vi "Dashboard Main.vi"() -> ()   [LabVIEW 2015]
uses:
  <vilib>/Utility/miscctls.llb/LVRowAndColumnTypeDef.ctl
  <vilib>/event_ctls.llb/eventvkey.ctl
  <vilib>/Rock Robotics/WPI/Dashboard/WPI_DashboardLogging Global.vi
  <vilib>/Rock Robotics/Network Tables/NT Read Numeric Array.vi
  <vilib>/Utility/config.llb/Write Key (String).vi
  <vilib>/Utility/config.llb/Write Key (I32).vi
  <vilib>/Utility/config.llb/NI_LVConfig.lvlib
panel:
  in  "TCP":refnum<k5>
  in  "Rec Mode":enum32{"Stop", "Record", "Playback"}(radio)
  in  "Vision":u16(ring) items=["Camera Off", "USB Camera SW", "USB Camera HW", "IP Camera"]
  out "Camera IP":string
  out "Image Message":string="Timeout in Camera Communications"
  in  "Dashboard Tab":T1(tab)
  out "String":string
  in  "Select Auto":string(combo)
  out "NT Connection":bool
  in  "Camera Settings":T2={"Frame Rate"=30, "Compression"=30, "Size"=1} {"Frame Rate" scale=1.0..30.0; "Size" items=["640x480", "320x240", "160x120"]}
  out "MotorChart R":cluster{"Numeric":dbl, "Numeric":dbl}(graph)
  out "MotorChart L":T3(graph)
  out "MotorSliders R":cluster{"MotorSlide1":dbl, "MotorSlide2":dbl} {"MotorSlide2" scale=-1.0..1.0 scale format="%#_2e"; "MotorSlide1" scale=-1.0..1.0 scale format="%#_2e"}
  out "MotorSliders L":T4 {"MotorSlide4 2" scale=0.0..14.0 scale format="%#_2e"; "MotorSlide2" scale=-1.0..1.0 scale format="%#_2e"; "MotorSlide1" scale=-1.0..1.0 scale format="%#_2e"}
  out "Gyro":dbl(knob) scale=0.0..360.0
  out "JS1 Z":dbl(slide) scale=-1.0..1.0 scale format="%#_2e"
  out "JS1 Graph":cluster{"X":dbl, "Y":dbl}[](graph)
  out "JS1 Buttons":T5
  out "JS2 Z":dbl(slide) scale=-1.0..1.0 scale format="%#_2e"
  out "JS2 Graph":cluster{"X":dbl, "Y":dbl}[](graph)
  out "JS2 Buttons":T5
  out "Mode":T6(ring)=enum."Auto Disabled"
  in  "DB Camera Config":bool
  out "fps":dbl format="%#.1g"
  out "Mbps":dbl format="%#.1g"
  out "Mbps LED":bool
  in  "Numeric":dbl
  in  "DB/String 9":string
  in  "DB/String 8":string
  in  "DB/String 7":string
  in  "DB/String 6":string
  in  "DB/String 5":string
  in  "DB/String 4":string
  in  "DB/String 3":string
  in  "DB/String 2":string
  in  "DB/String 1":string
  in  "DB/String 0":string
  in  "DB/Slider 0":dbl(slide) scale=0.0..5.0
  in  "DB/Slider 1":dbl(slide) scale=0.0..5.0
  in  "DB/Slider 2":dbl(slide) scale=0.0..5.0
  in  "DB/Slider 3":dbl(slide) scale=0.0..5.0
  out "DB/LED 3":bool
  out "DB/LED 2":bool
  out "DB/LED 1":bool
  out "DB/LED 0":bool
  in  "DB/Button 3":bool
  in  "DB/Button 2":bool
  in  "DB/Button 1":bool
  in  "DB/Button 0":bool caption="New Name"
  out "Gyro":dbl
  out "Sonar":dbl
  out "Gyro 2":dbl
  in  "Test Slider":dbl(slide) scale=0.0..100.0 scale format="%#_3g"
  in  "On/Off":bool caption="Solenoid"
  in  "Test Name":u16(ring) items=["Select the test to run..."]
  in  "Test Tree":string(tree)
  in  "Motor":cluster{"Value":dbl, "Enable":bool} {"Value" scale=-1.0..1.0 scale format="%#_3g"}
  out "Progress":T7 {"Test Progress" scale=0.0..100.0}
  in  "Rev/Fwd":cluster{"Forward":bool, "Reverse":bool}
  in  "Test Ring":u16(ring) items=["Monochrome", "Color"]
  out "Cmd Status":string
  in  "Execute Command":bool
  in  "Command Params":string[][](table)
  in  "Command Selection":i32(listbox)
  in  "CheckList":i32(listbox)
  out "Tree":string(tree)
  out "Camera Image":T8(plugin-control)
  out "Background":bool
  # "Left"
  # "Front"
  # "Right"
  # "Battery"
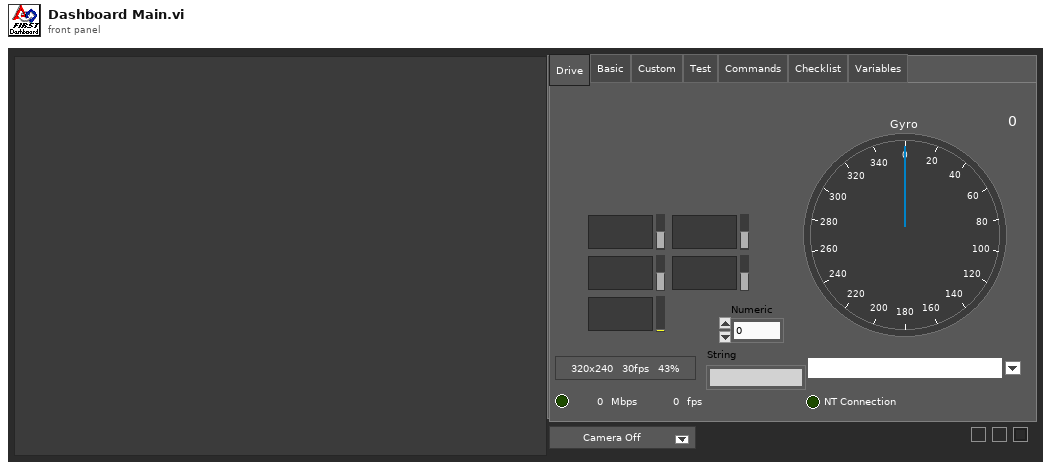
[diagram p1: front panel]
types:
  T1 = enum32{"Drive", "Basic", "Custom", "Test", "Commands", "Checklist", "Variables"}
  T2 = cluster{"Frame Rate":i32, "Compression":i32, "Size":u16}
  T3 = cluster{"Numeric":dbl, "Numeric":dbl, "Battery V":dbl}
  T4 = cluster{"MotorSlide1":dbl, "MotorSlide2":dbl, "MotorSlide4 2":dbl}
  T5 = cluster{bool, bool, bool, bool, bool, bool, bool, bool, bool, bool, bool, bool}
  T6 = enum8{"Tele-Op Disabled", "Tele-Op Enabled", "Auto Disabled", "Auto Enabled", "Test Disabled", "Test Enabled", "Disconnected", "No Code", "E-Stop"}
  T7 = cluster{"Test Progress":u8, "Test Progress Text":string}
  T8 = typedef "IMAQ Image.ctl" = refnum<image>
  T9 = cluster{"IDs":cluster{"RPC field ID":u16, "Unique ID":u16}, "String":string}
  T10 = enum32{"Drive", "Basic", "Custom", "Test", "Checklist", "Variables"}
  T11 = typedef "Image Type" = u32
  T12 = cluster{"Camera Image":refnum<vi>, "Dashboard Tab":refnum<vi>, "Background":refnum<vi>, "Vision":refnum<vi>, "Rec Mode":refnum<vi>, "Test Slider":refnum<vi>, "On/Off ":refnum<vi>, "Test Ring":refnum<vi>, "Rev/Fwd":refnum<vi>, "Test Name":refnum<vi>, "Motor":refnum<vi>, "Progress":refnum<vi>, "CheckList":refnum<vi>, "Tree":refnum<vi>, "Test Tree":refnum<vi>, "Command Params":refnum<vi>, "Command Selection":refnum<vi>, "Execute Command":refnum<vi>, "Cmd Status":refnum<vi>}
  T13 = cluster{"Error Strings":string, "Disable Counts":cluster{u16, u16}, "Rail Faults":cluster{u16, u16, u16}, "Robot IP":string, "DB Mode":u8, "Event Info":cluster{"Name":string, "Type":u8, "Number":u16, "Replay":u8}, "Camera Addr":string}
  T14 = cluster{"Storage":cluster{"Disk Free":u64, "RAM Block":u32, "RAM free":u32}, "CPU Utilization":cluster{"CPU % ISR":sgl, "CPU % Time Crit":sgl, "CPU % Timed Str":sgl, "CPU % High":sgl, "CPU % Above":sgl, "CPU % Normal":sgl, "CPU % Low":sgl}, "CAN":cluster{"% Bus Utilization":sgl, "Bus Off Cnt":u32, "TX_FIFO Full Cnt":u32, "Receive Error Cnt":u8, "Transmit Error Cnt":u8}, "HID":cluster{"HID Outputs":u32, "Rumble Low":u16, "Rumble High":u16}[]}
  T15 = cluster{"Status bits":cluster{"Test Mode":bool, "Autonomous":bool, "Enabled":bool, "Code Start":bool, "Brownout":bool, "Reserved 2":bool, "Reserved 3":bool, "E-Stop":bool}, "Code Trace":cluster{"Disabled":bool, "TeleOp":bool, "Auto":bool, "Test":bool}, "Controller Type":enum16{"unknown", "cRIO", "roboRio"}, "Code?":enum16{"unknown", "noCode", "code"}, "Battery V":dbl}
  T16 = cluster{"Control Bits":cluster{"TestMode":bool, "Autonomous":bool, "Enabled":bool, "FMS Present":bool, bool, bool, bool, "E-Stop":bool}, "Team Station ":u8, "Countdown":sgl, "Joystick Values":cluster{"Axes":dbl[], "Buttons":bool[], "POVs":i16[]}[]}
  T17 = cluster{"Axes":dbl[], "Buttons":bool[], "POVs":i16[]}[]
  T18 = cluster{"Axes":dbl[], "Buttons":bool[], "POVs":i16[]}
  T19 = cluster{"Buttons[0]":bool, "Buttons[1]":bool, "Buttons[2]":bool, "Buttons[3]":bool, "Buttons[4]":bool, "Buttons[5]":bool, "Buttons[6]":bool, "Buttons[7]":bool, "Buttons[8]":bool, "Buttons[9]":bool, "Buttons[10]":bool, "Buttons[11]":bool}
  T20 = cluster{"Desired Font (Application)":enum16{"User-specified Font", "Application Font", "System Font", "Dialog Font"}, "[User-specified Font]":cluster{"Font Name":string, "Size":i16, "Strikeout?":bool, "Italic?":bool, "Underline?":bool, "Outline?":bool, "Shadow?":bool, "Bold?":bool, "Rotation Angle":dbl}, "Horizontal Alignment":i16, "Vertical Alignment":i16}
  T21 = typedef "NI_LVConfig.lvlib/Config Data RefNum.ctl" = refnum<k1>
  T22 = cluster{"Operation":enum16{"Update", "Clear"}, "Color Box":u32}[]
  T23 = typedef "eventvkey.ctl" = enum16{"ASCII", "Enter", "Return", "Shift", "Ctrl", "Alt", "Cmd", "Opt", "Caps", "NumLock", "Clear", "Break", "Up", "Down", "Left", "Right", "Insert", "Delete", "Home", "End", "PageUp", "PageDown", "Escape", "Help", "Pause", "ScrollLock", "F1", "F2", "F3", "F4", "F5", "F6", "F7", "F8", "F9", "F10", "F11", "F12", "F13", "F14", "F15", "F16", "F17", "F18", "F19", "F20", "F21", "F22", "F23", "F24", "Play", "VolumeUp", "VolumeDown", "Mute", "Two Byte Char"}
  T24 = cluster{"Image Size":bool, "Image Type":bool, "Pixel Value":bool, "ROI Information":bool, "Zoom Factor":bool}
  T25 = enum8{"Enabled", "Disabled", "Disabled and Grayed Out"}
  T26 = cluster{"Operation":enum16{"Update", "Clear"}, "Color Box":u32}
  T27 = typedef "LVRowAndColumnTypeDef.ctl" = cluster{"Row":i32, "Column":i32}
  T28 = cluster{"Shift":bool, "Ctrl":bool, "Alt":bool, "Cmd":bool, "Opt":bool}
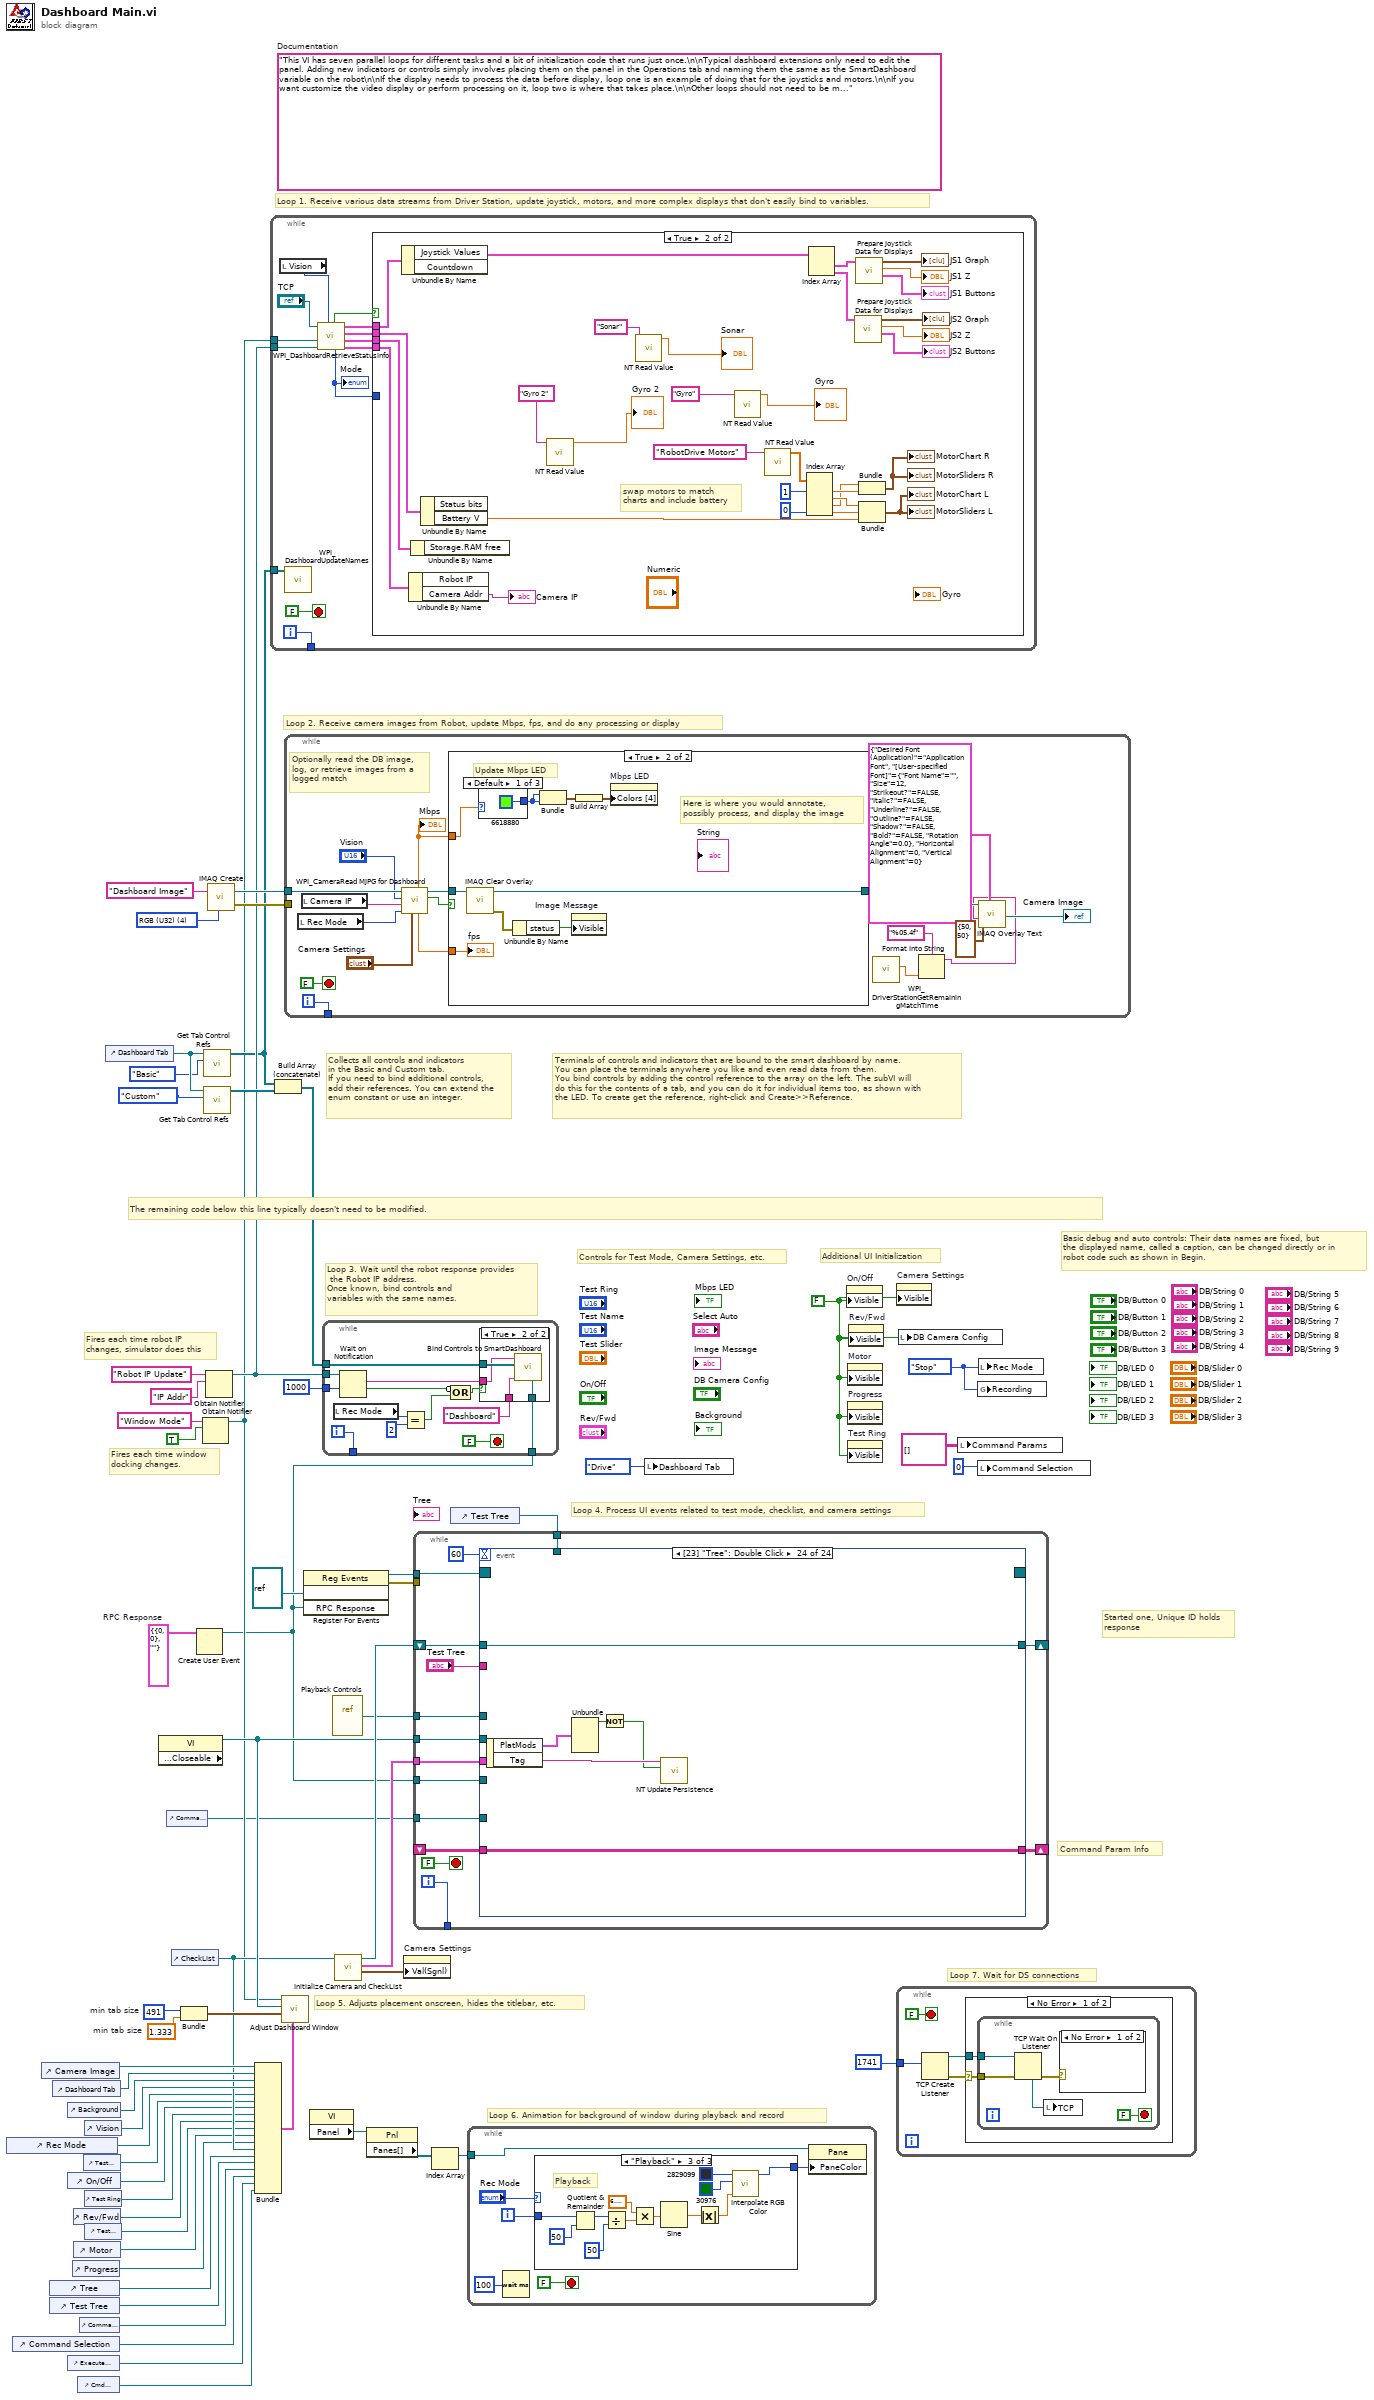
[diagram p0: block diagram]
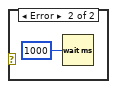
[diagram p2: hidden frame]
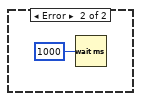
[diagram p3: hidden frame]
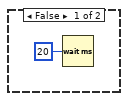
[diagram p4: hidden frame]
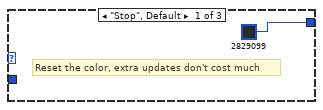
[diagram p5: hidden frame]
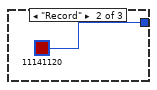
[diagram p6: hidden frame]
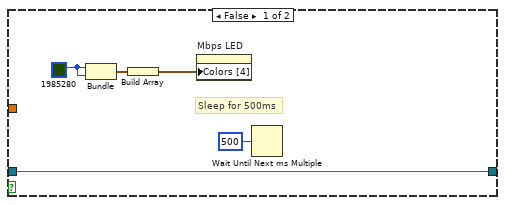
[diagram p8: hidden frame]
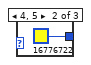
[diagram p9: hidden frame]
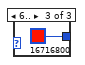
[diagram p10: hidden frame]
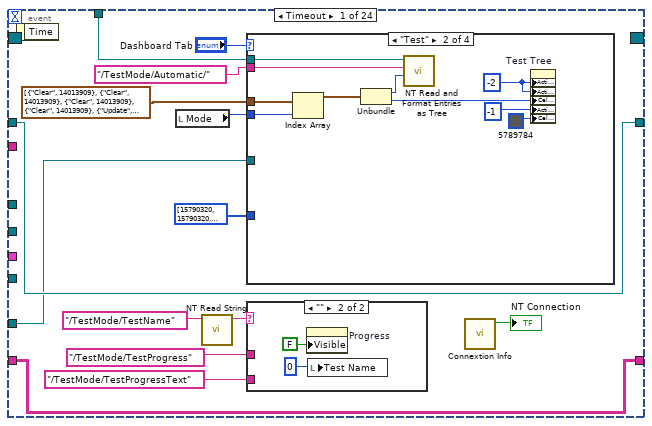
[diagram p11: hidden frame]
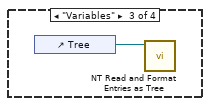
[diagram p13: hidden frame]
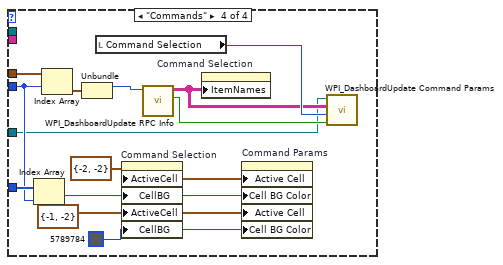
[diagram p14: hidden frame]
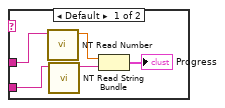
[diagram p15: hidden frame]
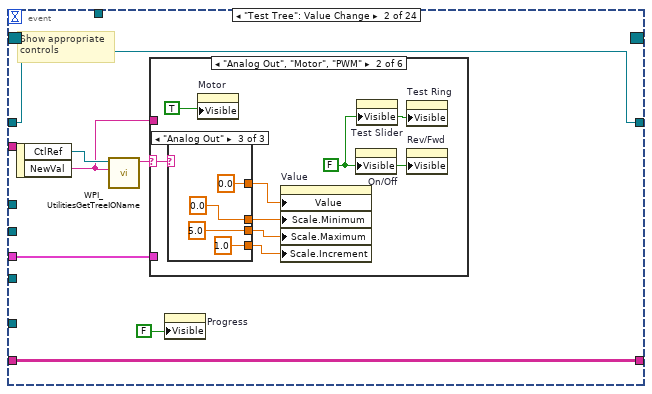
[diagram p16: hidden frame]
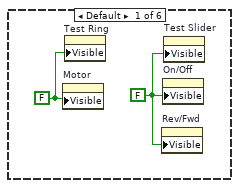
[diagram p17: hidden frame]
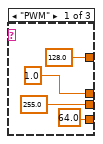
[diagram p18: hidden frame]
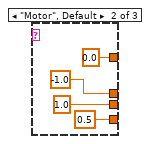
[diagram p19: hidden frame]
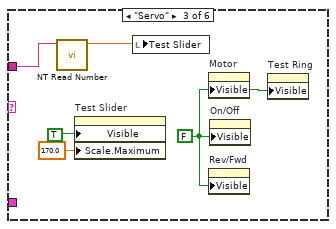
[diagram p20: hidden frame]
diagram:
  w7 = T9 {"IDs"={"RPC field ID"=0, "Unique ID"=0}, "String"=""}  # RPC Response
  w33 = 491  # min tab size
  w32 = 1.333  # min tab size
  w41 = enum32{"Stop", "Record", "Playback"}."Stop" ("Rec Mode")
  w15 = FALSE ("Visible")
  (unwired) "This VI has seven parallel loops for different tasks and a bit of initialization code that runs just once.\n\nTypical dashboard extensions only need to edit the panel. Adding new indicators or controls simply involves placing them on the panel in the Operations tab and naming them the same as the SmartDashboard variable on the robot\n\nIf the display needs to process the data before display, loop one is an example of doing that for the joysticks and motors.\n\nIf you want customize the video display or perform processing on it, loop two is where that takes place.\n\nOther loops should not need to be modified. They are pretty standard, and document the task they perform."  # Documentation
  w61 = T11 4 items=["Grayscale (U8)", "Grayscale (I16)", "Grayscale (SGL)", "Complex (CSG)", "RGB (U32)", "HSL (U32)", "RGB (U64)"] ("Image Type")
  # "Command Param Info"
  # "Started one, Unique ID holds\nresponse"
  # "Loop 7. Wait for DS connections"
  # "Basic debug and auto controls: Their data names are fixed, but\nthe displayed name, called a caption, can be changed directly or in\nrobot code such as shown in Begin."
  # "Controls for Test Mode, Camera Settings, etc."
  # "Additional UI Initialization"
  # "Loop 6. Animation for background of window during playback and record"
  # "Fires each time robot IP\nchanges, simulator does this"
  # "Fires each time window\ndocking changes."
  # "Collects all controls and indicators\nin the Basic and Custom tab.\nIf you need to bind additional controls,\nadd their references. You can extend the\nenum constant or use an integer."
  # "The remaining code below this line typically doesn't need to be modified."
  # "Loop 4. Process UI events related to test mode, checklist, and camera settings"
  # "Terminals of controls and indicators that are bound to the smart dashboard by name.\nYou can place the terminals anywhere you like and even read data from them.\nYou bind controls by adding the control reference to the array on the left. The subVI will\ndo this for the contents of a tab, and you can do it for individual items too, as shown with\nthe LED. To create get the reference, right-click and Create>>Reference."
  # "Loop 3. Wait until the robot response provides\n the Robot IP address.\nOnce known, bind controls and\nvariables with the same names."
  # "Loop 5. Adjusts placement onscreen, hides the titlebar, etc."
  # "Loop 1. Receive various data streams from Driver Station, update joystick, motors, and more complex displays that don't easily bind to variables."
  # "Loop 2. Receive camera images from Robot, update Mbps, fps, and do any processing or display"
  n1 = control-ref of="Rec Mode"() -> (w21:refnum<vi>)
  n2 = control-ref of="Command Selection"() -> (w6:refnum<vi>)
  n3 = control-ref of="Camera Image"() -> (w36:refnum<vi>)
  n4 = control-ref of="Tree"() -> (w25:refnum<vi>)
  n5 = control-ref of="Test Tree"() -> (w24:refnum<vi>)
  n6 = control-ref of="Dashboard Tab"() -> (w35:refnum<vi>)
  n7 = control-ref of="Execute Command"() -> (w8:refnum<vi>)
  n8 = control-ref of="Background"() -> (w30:refnum<vi>)
  n9 = control-ref of="On/Off"() -> (w19:refnum<vi>)
  n10 = control-ref of="Progress"() -> (w16:refnum<vi>)
  n11 = control-ref of="Rev/Fwd"() -> (w17:refnum<vi>)
  n12 = control-ref of="Motor"() -> (w22:refnum<vi>)
  n13 = control-ref of="Cmd Status"() -> (w2:refnum<vi>)
  n14 = control-ref of="Command Params"() -> (w9:refnum<vi>)
  n15 = control-ref of="Test Slider"() -> (w20:refnum<vi>)
  n16 = control-ref of="Vision"() -> (w34:refnum<vi>)
  n17 = control-ref of="Test Ring"() -> (w18:refnum<vi>)
  n18 = control-ref of="Test Name"() -> (w23:refnum<vi>)
  n19 = control-ref of="Dashboard Tab"() -> (w39:refnum<vi>)
  n20 = property class="VI" props=["Front Panel.Closeable"]() -> (reference out=w40:refnum<vi>)  [unwired: 2 in, 2 out]
  n21 = control-ref of="Command Params"() -> (w1:refnum<vi>)
  n22 = control-ref of="CheckList"() -> (w26:refnum<vi>)
  n23 = Bundle("min tab size"=w33, "min tab size"=w32) -> (w31:cluster{"min tab size":i32, "min tab size":dbl})  [unwired: 1 in]
  n24 = Create User Event(user event datatype=w7) -> (user event=w3:refnum<user-event>)  [unwired: 1 in, 1 out]
  n25 = Obtain Notifier(name (unnamed)="Window Mode", notification data type=TRUE) -> (notifier out=w12:refnum<notifier>)  [unwired: 2 in, 2 out]
  n26 = call <vilib>:"Get Tab Control Refs.vi"("Page Index"=T10."Basic" ("Dashboard Tab"), "TabControl in"=w39) -> ("ControlsOnPage"=w13:refnum<vi>[])  [unwired: 9 in]
  n27 = call <vilib>:"Get Tab Control Refs.vi"("Page Index"=T10."Custom" ("Dashboard Tab"), "TabControl in"=w39) -> ("ControlsOnPage"=w38:refnum<vi>[])  [unwired: 9 in]
  n28 = Obtain Notifier(name (unnamed)="Robot IP Update", notification data type="IP Addr" ("name (unnamed)")) -> (notifier out=w14:refnum<notifier>)  [unwired: 2 in, 2 out]
  n29 = call "IMAQ Create"("Image Name"="Dashboard Image", "Image Type"=w61) -> ("New Image"=w59:T8, "error out"=w58:errorcluster)  [unwired: 2 in, 1 out]
  n30 = Bundle("Camera Image"=w36, "Dashboard Tab"=w35, "Background"=w30, "Vision"=w34, "Rec Mode"=w21, "Test Slider"=w20, "On/Off"=w19, "Test Ring"=w18, "Rev/Fwd"=w17, "Test Name"=w23, "Motor"=w22, "Progress"=w16, "CheckList"=w26, "Tree"=w25, "Test Tree"=w24, "Command Params"=w9, "Command Selection"=w6, "Execute Command"=w8, "Cmd Status"=w2) -> (w27:T12)  [unwired: 1 in]
  n31 = while {
    tunnel: [w73] -> _
    tunnel: w14 -> [w67]
    tunnel: w13 -> [w66]
    tunnel: w12 -> [w62]
    i -> [w73]
    stop <- FALSE stop-if-true
    n32 = local read "Vision"() -> (w64:u16)
    n33 = call <vilib>:"WPI_DashboardUpdateNames.vi"("Controls on Tab"=w66) -> ()  [unwired: 11 in]
    n34 = call <vilib>:"WPI_DashboardRetrieveStatusInfo.vi"("Vision"=w64, "Binding Refnum"=w67, "Window Mode Notifier"=w62, "TCP Cnx"="TCP") -> ("Power and Errors"=w68:T13, "Robot Metrics"=w71:T14, "Status Info"=w72:T15, "Control Info"=w69:T16, "Robot Mode"=w65:T6, "Process?"=w70:bool)  [unwired: 2 in]
    "Mode" <- w65
    n35 = case shown="True" w70 {
      tunnel: w72 -> [_ w106]
      tunnel: w71 -> [_ w105]
      tunnel: w69 -> [_ w104]
      tunnel: w68 -> [_ w103]
      tunnel: w65 -> [_ _]
      frame False {
        n36 = Wait (ms)(milliseconds to wait=u32 20) -> ()  [unwired: 1 out]
      }
      frame True {
        # "swap motors to match\ncharts and include battery"
        n37 = Unbundle By Name(w104) -> ("Joystick Values"=w93:T17)  [unwired: 1 out]
        n38 = Unbundle By Name(w103) -> ("Camera Addr"=→"Camera IP":string)  [unwired: 1 out]
        n39 = Unbundle By Name(w105) -> ()  [unwired: 1 out]
        n40 = Unbundle By Name(w106) -> ("Battery V"=w94:dbl)  [unwired: 1 out]
        n41 = call-poly <vilib>:"NT Read Value.vi"("Name"="Gyro 2") -> ("Numeric"=→"Gyro 2":dbl)  [unwired: 9 in, 1 out]
        n42 = call-poly <vilib>:"NT Read Value.vi"("Name"="Sonar") -> ("Numeric"=→"Sonar":dbl)  [unwired: 9 in, 1 out]
        n43 = call-poly <vilib>:"NT Read Value.vi"("Name"="Gyro") -> ("Numeric"=→"Gyro":dbl)  [unwired: 9 in, 1 out]
        n44 = call-poly <vilib>:"NT Read Value.vi"("Name"="RobotDrive Motors") -> ("Numeric Array"=w82:dbl[])  [unwired: 9 in, 1 out]
        n45 = Index Array(array=w82, index #1=1, index #4=0) -> (element #1=w98:dbl, element #2=w99:dbl, element #3=w97:dbl, element #4=w102:dbl)  [unwired: 2 in]
        n46 = Index Array(array=w93) -> (element #1=w92:T18, element #2=w87:T18)  [unwired: 2 in]
        n47 = call "Prepare Joystick Data for Displays.vi"("Joystick Values"=w87) -> ("Buttons"=→"JS2 Buttons":T19, "Z Axis"=→"JS2 Z":dbl, "Cartesian Data"=→"JS2 Graph":cluster{"X axis":dbl, "X axis":dbl}[])  [unwired: 8 in]
        n48 = call "Prepare Joystick Data for Displays.vi"("Joystick Values"=w92) -> ("Buttons"=→"JS1 Buttons":T19, "Z Axis"=→"JS1 Z":dbl, "Cartesian Data"=→"JS1 Graph":cluster{"X axis":dbl, "X axis":dbl}[])  [unwired: 8 in]
        n49 = Bundle("Numeric"=w97, "Numeric"=w98) -> (→"MotorChart R" →"MotorSliders R":cluster{"Numeric":dbl, "Numeric":dbl})  [unwired: 1 in]
        n50 = Bundle("Numeric"=w99, "Numeric"=w102, "Battery V"=w94) -> (→"MotorChart L" →"MotorSliders L":T3)  [unwired: 1 in]
      }
    }
  }
  n51 = Build Array (concatenate)(w13, w38) -> (w37:refnum<vi>[])
  n52 = call "Adjust Dashboard Window.vi"("Sizing Refnums"=w27, "Size Constraints"=w31, "VI"=w40, "WIn Mode"=w12) -> ()  [unwired: 8 in]
  n53 = while {
    tunnel: w59 -> [w122]
    tunnel: w58 -> [_]
    tunnel: [w123] -> _
    i -> [w123]
    stop <- FALSE stop-if-true
    # "Optionally read the DB image,\nlog, or retrieve images from a\nlogged match"
    n54 = local read "Rec Mode"() -> (w117:enum32{"Stop", "Record", "Playback"})
    n55 = local read "Camera IP"() -> (w115:string)
    n56 = call <vilib>:"WPI_CameraRead MJPG for Dashboard.vi"("Camera Settings"="Camera Settings", "Rec Mode"=w117, "Camera IP"=w115, "Camera Mode"="Vision", "Refnum in"=w122) -> ("Active"=w120:bool, "Refnum out"=w121:T8, "FPS"=w119:dbl, "Bandwidth (Mbps)"=w114:dbl)  [unwired: 3 in]
    "Mbps" <- w114
    n57 = case shown="True" w120 {
      tunnel: w121 -> [w125 w133]
      tunnel: w114 -> [_ w132]
      tunnel: w119 -> [_ w131]
      tunnel: [w125 w130] -> w113
      frame False {
        w126 = u32 1985280 ("Color Box")
        # "Sleep for 500ms"
        n58 = Bundle("Color Box"=w126, "Color Box"=w126) -> (w128:cluster{"Color Box":u32, "Color Box":u32})  [unwired: 1 out]
        n59 = Build Array(w128) -> (w127:cluster{"Color Box":u32, "Color Box":u32}[])
        n60 = property on="Mbps LED" class="Bool (strict)"("Colors [4]"=w127) -> ()  [unwired: 2 in, 2 out]
        n61 = Wait Until Next ms Multiple(millisecond multiple=u32 500) -> ()  [unwired: 1 out]
      }
      frame True {
        # "Here is where you would annotate,\npossibly process, and display the image"
        # "Update Mbps LED"
        n62 = call "IMAQ Clear Overlay"("Image"=w133) -> ("error out"=w137:errorcluster, "Image Out"=w130:T8)  [unwired: 2 in, 7 out]
        n63 = case shown="Default" w132 {
          tunnel: [u32 6618880 ("Color Box") u32 16776722 ("Color Box") u32 16716800 ("Color Box")] -> w134
          frame Default {
          }
          frame 4, 5 {
          }
          frame 6.. {
          }
        }
        n64 = Unbundle By Name(w137) -> ("status"=w138:bool)
        n65 = Bundle("Color Box"=w134, "Color Box"=w134) -> (w136:cluster{"Color Box":u32, "Color Box":u32})  [unwired: 1 out]
        n66 = property on="Image Message" class="Str"("Visible"=w138) -> ()  [unwired: 2 in, 2 out]
        n67 = Build Array(w136) -> (w135:cluster{"Color Box":u32, "Color Box":u32}[])
        n68 = property on="Mbps LED" class="Bool (strict)"("Colors [4]"=w135) -> ()  [unwired: 2 in, 2 out]
        "fps" <- w131
      }
    }
    n69 = call <vilib>:"WPI_DriverStationGetRemainingMatchTime.vi"() -> ("Match Time(s)"=w109:sgl)  [unwired: 10 in, 1 out]
    n70 = Format Into String(format string="%05.4f", w109) -> (resulting string=w108:string)  [unwired: 2 in, 1 out]
    n71 = call "IMAQ Overlay Text"("Font, Size & Style"=T20 {"Desired Font (Application)"=enum."Application Font", "[User-specified Font]"={"Font Name"="", "Size"=12, "Strikeout?"=FALSE, "Italic?"=FALSE, "Underline?"=FALSE, "Outline?"=FALSE, "Shadow?"=FALSE, "Bold?"=FALSE, "Rotation Angle"=0.0}, "Horizontal Alignment"=0, "Vertical Alignment"=0}, "String"=w108, "Origin"=cluster{"X":i32, "Y":i32} {"X"=50, "Y"=50}, "Image"=w113) -> ("Image Out"=→"Camera Image":T8)  [unwired: 6 in, 1 out]
  }
  n72 = register-events(refnum<vi> refnum, w3) -> (reference out=w45:refnum<event-registration>, error out=w44:errorcluster)  [unwired: 2 in]
  n73 = property class="VI"() -> ("Panel"=w48:refnum<vi>)  [unwired: 2 in, 2 out]
  n74 = while {
    tunnel: w37 -> [w154]
    tunnel: w14 -> [w152]
    tunnel: [w150] -> _
    tunnel: u32 1000 ("milliseconds to wait") -> [w149]
    tunnel: w3 -> [w142]
    i -> [w150]
    stop <- FALSE stop-if-true
    n75 = local read "Rec Mode"() -> (w145:enum32{"Stop", "Record", "Playback"})
    n76 = Wait on Notification(notifier=w152, timeout in ms (-1)=w149) -> (notification=w151:string, timed out?=w147:bool)  [unwired: 2 in, 2 out]
    n77 = Equal?(x=w145, y=u16 2 ("Rec Mode")) -> (x = y?=w146:bool)
    n78 = Compound Arithmetic op=OR(invert w147, w146) -> (w148:bool)
    n79 = case shown="True" w148 {
      tunnel: w154 -> [_ w158]
      tunnel: w151 -> [_ w157]
      tunnel: "Dashboard" -> [_ w156]
      tunnel: w142 -> [_ w155]
      frame False {
      }
      frame True {
        n80 = call <vilib>:"Bind Controls to SmartDashboard.vi"("RPC ref"=w155, "Client Name"=w156, "Bound Control Refs"=w158, "Server IP Address"=w157) -> ()  [unwired: 8 in]
      }
    }
  }
  n81 = vi-ref "Playback Controls.vi"() -> (w46:refnum<vi>)
  n82 = call "Initialize Camera and CheckList.vi"("ListBox in"=w26) -> ("Cluster"=w52:cluster{"value":i32, "value":i32, "index":i32}, "Array"=w53:cluster{string[]}[], "File Refnum"=w51:T21)  [unwired: 8 in]
  n83 = property class="Pnl"(reference=w48) -> ("Panes[]"=w49:refnum<vi>[])  [unwired: 1 in, 2 out]
  n84 = property on="Camera Settings" class="Clust (strict)"("Val(Sgnl)"=w52) -> ()  [unwired: 2 in, 2 out]
  n85 = Index Array(array=w49) -> (element=w47:refnum<vi>)  [unwired: 1 in]
  n86 = control-ref of="Test Tree"() -> (w50:refnum<vi>)
  n87 = while {
    tunnel: w53 -> [w170]
    shift-right: [w169] -> _
    shift-left: w51 -> [w168]
    tunnel: [w167] -> _
    tunnel: w50 -> [w166]
    tunnel: w46 -> [w165]
    tunnel: w45 -> [w164]
    tunnel: w44 -> [_]
    tunnel: w40 -> [w163]
    tunnel: w3 -> [w162]
    tunnel: w1 -> [w161]
    shift-right: [w160] -> _
    shift-left: _ -> [w159]
    i -> [w167]
    stop <- FALSE stop-if-true
    n88 = event shown="[23] \"Tree\": Double Click" {
      selector: w164 -> [_ _ _ _ _ _ _ _ _ _ _ _ _ _ _ _ _ _ _ _ _ _ _ _]
      dyn-events: [_ _ _ _ _ _ _ _ _ _ _ _ _ _ _ _ _ _ w479 _ _ _ _ _] -> _
      timeout: u32 60 ("milliseconds to wait") -> [_ _ _ _ _ _ _ _ _ _ _ _ _ _ _ _ _ _ _ _ _ _ _ _]
      tunnel: w166 -> [w183 _ _ _ _ _ _ _ _ _ _ _ _ _ _ _ _ _ _ _ _ _ _ _]
      tunnel: "Test Tree" -> [_ _ _ _ _ _ _ _ _ _ _ _ _ w442 w451 w454 w459 w468 _ _ _ _ _ _]
      tunnel: w170 -> [_ w221 _ _ _ _ _ _ _ _ _ w404 w435 _ _ _ _ _ _ _ _ _ _ _]
      tunnel: [w180 w220 w324 w330 w340 w344 w350 w362 w370 w376 w389 w403 w428 w441 w449 w453 w458 w467 w481 w497 w499 w507 w518 w523] -> w169
      tunnel: w168 -> [w180 w220 w324 w330 w340 w344 w350 w362 w370 w376 w389 w402 w428 w441 w449 w453 w458 w467 w481 w497 w499 w507 w518 w523]
      tunnel: w165 -> [_ _ _ _ _ _ _ _ _ _ _ _ _ _ _ _ _ _ w482 _ w502 _ _ _]
      tunnel: w163 -> [_ _ _ _ _ _ _ _ _ _ _ _ _ _ _ _ _ _ w477 _ _ _ _ _]
      tunnel: w162 -> [_ _ _ _ _ _ _ _ _ _ _ _ _ _ _ _ _ _ w473 _ _ _ _ _]
      tunnel: w161 -> [w175 _ _ _ _ _ w348 _ _ _ _ _ _ _ _ _ _ _ _ _ _ _ _ _]
      tunnel: [w174 w219 w323 w329 w339 w345 w346 w356 w367 w375 w388 w401 w427 w440 w448 w452 w457 w466 w472 w495 w498 w503 w511 w524] -> w160
      tunnel: w159 -> [w174 w219 w323 w329 w339 w345 w346 _ _ w375 w388 w401 w427 w440 w448 w452 w457 w466 w472 w495 w498 w503 w511 w524]
      event Timeout {
        n89 = event-data() -> ()  [unwired: 1 in, 1 out]
        n90 = local read "Mode"() -> (w177:T6)
        n91 = call <vilib>:"NT Read String.vi"("Name"="/TestMode/TestName") -> ("String"=w186:string)  [unwired: 9 in, 1 out]
        n92 = case shown="\"Test\"" "Dashboard Tab" {
          tunnel: w183 -> [_ w197 _ _]
          tunnel: "/TestMode/Automatic/" ("Name Pattern") -> [_ w196 _ _]
          tunnel: T22 [{"Operation"=enum."Clear", "Color Box"=14013909}, {"Operation"=enum."Clear", "Color Box"=14013909}, {"Operation"=enum."Clear", "Color Box"=14013909}, {"Operation"=enum."Clear", "Color Box"=14013909}, {"Operation"=enum."Update", "Color Box"=14013909}, {"Operation"=enum."Update", "Color Box"=16777215}, {"Operation"=enum."Clear", "Color Box"=14013909}, {"Operation"=enum."Clear", "Color Box"=14013909}, {"Operation"=enum."Clear", "Color Box"=14013909}] -> [_ w189 _ w206]
          tunnel: w177 -> [_ w188 _ w205]
          tunnel: u32[] [15790320, 15790320, 15790320, 15790320, 16777215, 16777215, 15790320, 15790320, 15790320] -> [_ _ _ w211]
          tunnel: w175 -> [_ _ _ w199]
          frame "Custom", Default {
          }
          frame "Test" {
            w195 = -2 ("Active Item:Row Number")
            n93 = Index Array(array=w189, index=w188) -> (element=w190:T26)
            n94 = Unbundle(w190) -> ("Operation"=w191:enum16{"Update", "Clear"}, "Color Box"=w192:u32)
            n95 = call <vilib>:"NT Read and Format Entries as Tree.vi"("Operation"=w191, "Name Pattern"=w196, "Tree Refnum"=w197) -> ()  [unwired: 7 in, 2 out]
            n96 = property on="Test Tree" class="Tree (strict)"("Active Item Row Number"=w195, "ActiveColNum"=w195, "CellBG"=w192, "Active Item Row Number"=-1 ("Active Item:Row Number"), "CellBG"=u32 5789784 ("Color Box")) -> ()  [unwired: 2 in, 2 out]
          }
          frame "Variables" {
            n97 = control-ref of="Tree"() -> (w198:refnum<vi>)
            n98 = call <vilib>:"NT Read and Format Entries as Tree.vi"("Tree Refnum"=w198) -> ()  [unwired: 9 in, 2 out]
          }
          frame "Commands" {
            w207 = u32 5789784 ("Color Box")
            w208 = T27 {"Row"=-1, "Column"=-2} ("Active Cell:Active Cell")
            w210 = T27 {"Row"=-2, "Column"=-2} ("Active Cell:Active Cell")
            n99 = Index Array(array=w211, index=w205) -> (element=w209:u32)
            n100 = Index Array(array=w206, index=w205) -> (element=w204:T26)
            n101 = Unbundle(w204) -> ("Operation"=w203:enum16{"Update", "Clear"})  [unwired: 1 out]
            n102 = local read "Command Selection"() -> (w202:i32)
            n103 = property on="Command Selection" class="MCListbox (strict)"("ActiveCell"=w210, "CellBG"=w209, "ActiveCell"=w208, "CellBG"=w207) -> ()  [unwired: 2 in, 2 out]
            n104 = call <vilib>:"WPI_DashboardUpdate RPC Info.vi"("Operation"=w203) -> ("update"=w201:bool, "commands"=w200:string[][])  [unwired: 9 in]
            n105 = property on="Command Selection" class="MCListbox (strict)"("ItemNames"=w200) -> ()  [unwired: 2 in, 2 out]
            n106 = property on="Command Params" class="Tbl (strict)"("Active Cell"=w210, "Cell BG Color"=w209, "Active Cell"=w208, "Cell BG Color"=w207) -> ()  [unwired: 2 in, 2 out]
            n107 = call <vilib>:"WPI_DashboardUpdate Command Params.vi"("Update"=w201, "NewVal"=w202, "Commands"=w200, "Param Tbl"=w199) -> ()  [unwired: 7 in, 1 out]
          }
        }
        n108 = case shown="\"\"" w186 {
          tunnel: "/TestMode/TestProgress" ("Name") -> [w213 _]
          tunnel: "/TestMode/TestProgressText" ("Name") -> [w212 _]
          frame Default {
            n109 = call <vilib>:"NT Read Number.vi"("Name"=w213) -> ("Numeric"=w214:dbl)  [unwired: 9 in, 1 out]
            n110 = call <vilib>:"NT Read String.vi"("Name"=w212) -> ("String"=w215:string)  [unwired: 9 in, 1 out]
            n111 = Bundle("Numeric"=w214, "String"=w215) -> (→"Progress":cluster{"Numeric":dbl, "String":string})  [unwired: 1 in]
          }
          frame "" {
            n112 = property on="Progress" class="Clust (strict)"("Visible"=FALSE) -> ()  [unwired: 2 in, 2 out]
            n113 = local write "Test Name"(u16 0) -> ()
          }
        }
        n114 = call <vilib>:"Connextion Info.vi"() -> ("Connected"=→"NT Connection":bool)  [unwired: 10 in, 1 out]
      }
      event "Test Tree": Value Change {
        # "Show appropriate\ncontrols"
        n115 = event-data() -> ("CtlRef"=w224:refnum<vi>, "NewVal"=w222:string)  [unwired: 1 in]
        n116 = call <vilib>:"WPI_UtilitiesGetTreeIOName.vi"("NewVal"=w222, "TreeControl in"=w224) -> ("I/O Name"=w225:string)  [unwired: 9 in]
        n117 = case shown="\"Analog Out\", \"Motor\", \"PWM\"" w225 {
          selector: w225 -> [_ w232 _ w254 w263 _]
          tunnel: w222 -> [_ _ w251 w253 _ w270]
          tunnel: w221 -> [_ _ _ _ _ w269]
          frame Default {
            w227 = FALSE ("Visible")
            w226 = FALSE ("Visible")
            n118 = property on="Motor" class="Clust (strict)"("Visible"=w226) -> ()  [unwired: 2 in, 2 out]
            n119 = property on="Test Ring" class="Ring (strict)"("Visible"=w226) -> ()  [unwired: 2 in, 2 out]
            n120 = property on="Rev/Fwd" class="Clust (strict)"("Visible"=w227) -> ()  [unwired: 2 in, 2 out]
            n121 = property on="On/Off" class="Bool (strict)"("Visible"=w227) -> ()  [unwired: 2 in, 2 out]
            n122 = property on="Test Slider" class="Slide (strict)"("Visible"=w227) -> ()  [unwired: 2 in, 2 out]
          }
          frame "Analog Out", "Motor", "PWM" {
            w233 = FALSE ("Visible")
            n123 = case shown="\"Analog Out\"" w232 {
              tunnel: [1.0 ("Value") -1.0 ("Value") 0.0 ("Value")] -> w231
              tunnel: [255.0 ("Value") 1.0 ("Value") 5.0 ("Value")] -> w230
              tunnel: [128.0 ("Value") 0.0 ("Value") 0.0 ("Value")] -> w229
              tunnel: [64.0 ("Value") 0.5 ("Value") 1.0 ("Value")] -> w228
              frame "PWM" {
              }
              frame "Motor", Default {
              }
              frame "Analog Out" {
              }
            }
            n124 = property on="Motor" class="Clust (strict)"("Visible"=TRUE) -> ()  [unwired: 2 in, 2 out]
            n125 = property on="Value" class="Slide (strict)"("Value"=w229, "Scale.Minimum"=w231, "Scale.Maximum"=w230, "Scale.Increment"=w228) -> ()  [unwired: 2 in, 2 out]
            n126 = property on="On/Off" class="Bool (strict)"("Visible"=w233) -> ()  [unwired: 2 in, 2 out]
            n127 = property on="Test Slider" class="Slide (strict)"("Visible"=w233) -> ()  [unwired: 2 in, 2 out]
            n128 = property on="Test Ring" class="Ring (strict)"("Visible"=w233) -> ()  [unwired: 2 in, 2 out]
            n129 = property on="Rev/Fwd" class="Clust (strict)"("Visible"=w233) -> ()  [unwired: 2 in, 2 out]
          }
          frame "Servo" {
            w249 = FALSE ("Visible")
            n130 = call <vilib>:"NT Read Number.vi"("Name"=w251) -> ("Numeric"=w250:dbl)  [unwired: 9 in, 1 out]
            n131 = property on="Test Slider" class="Slide (strict)"("Visible"=TRUE, "Scale.Maximum"=170.0 ("Scale.Range:Maximum")) -> ()  [unwired: 2 in, 2 out]
            n132 = local write "Test Slider"(w250) -> ()
            n133 = property on="Motor" class="Clust (strict)"("Visible"=w249) -> ()  [unwired: 2 in, 2 out]
            n134 = property on="Rev/Fwd" class="Clust (strict)"("Visible"=w249) -> ()  [unwired: 2 in, 2 out]
            n135 = property on="On/Off" class="Bool (strict)"("Visible"=w249) -> ()  [unwired: 2 in, 2 out]
            n136 = property on="Test Ring" class="Ring (strict)"("Visible"=w249) -> ()  [unwired: 2 in, 2 out]
          }
          frame "Relay", "Solenoid" {
            w252 = FALSE ("Visible")
            n137 = property on="Motor" class="Clust (strict)"("Visible"=w252) -> ()  [unwired: 2 in, 2 out]
            n138 = property on="Test Slider" class="Slide (strict)"("Visible"=w252) -> ()  [unwired: 2 in, 2 out]
            n139 = Search and Replace String(input string=w253, search string="/Value  **", replace string="/Direction") -> (result string=w259:string)  [unwired: 5 in, 3 out]
            n140 = property on="Test Ring" class="Ring (strict)"("Visible"=w252) -> ()  [unwired: 2 in, 2 out]
            n141 = call <vilib>:"NT Read String.vi"("Name"=w259) -> ("String"=w257:string)  [unwired: 9 in, 1 out]
            n142 = Equal?(x="Both directions", y=w257) -> (x = y?=w255:bool)
            n143 = Not(x=w255) -> (.not. x?=w256:bool)
            n144 = property on="Rev/Fwd" class="Clust (strict)"("Visible"=w255) -> ()  [unwired: 2 in, 2 out]
            n145 = property on="On/Off" class="Bool (strict)"("Visible"=w256, "Caption.Text"=w254) -> ()  [unwired: 2 in, 2 out]
          }
          frame "Compressor", "Digital Out" {
            w262 = FALSE ("Visible")
            # "Get direction and finish"
            n146 = property on="Motor" class="Clust (strict)"("Visible"=w262) -> ()  [unwired: 2 in, 2 out]
            n147 = property on="Test Slider" class="Slide (strict)"("Visible"=w262) -> ()  [unwired: 2 in, 2 out]
            n148 = property on="Test Ring" class="Ring (strict)"("Visible"=w262) -> ()  [unwired: 2 in, 2 out]
            n149 = property on="On/Off" class="Bool (strict)"("Visible"=TRUE, "Caption.Text"=w263) -> ()  [unwired: 2 in, 2 out]
            n150 = property on="Rev/Fwd" class="Clust (strict)"("Visible"=FALSE) -> ()  [unwired: 2 in, 2 out]
          }
          frame "Camera" {
            n151 = call <vilib>:"Get Last Path Segment.vi"("String in"=w270) -> ("String out"=w271:string)  [unwired: 10 in]
            n152 = property on="On/Off" class="Bool (strict)"("Visible"=FALSE) -> ()  [unwired: 2 in, 2 out]
            n153 = property on="Motor" class="Clust (strict)"("Visible"=FALSE) -> ()  [unwired: 2 in, 2 out]
            n154 = property on="Rev/Fwd" class="Clust (strict)"("Visible"=FALSE) -> ()  [unwired: 2 in, 2 out]
            n155 = case shown="\"White Balance  **\"" w271 {
              tunnel: w270 -> [w277 w286 w295 w304 w313 _ w319]
              tunnel: w269 -> [w275 w283 w292 w301 w310 _ _]
              frame "Size  **" {
                n156 = Index Array(array=w275) -> (element=w274:cluster{string[]})  [unwired: 1 in]
                n157 = call <vilib>:"NT Read String.vi"("Name"=w277) -> ("String"=w276:string)  [unwired: 9 in, 1 out]
                n158 = Unbundle(w274) -> (w272:string[])
                n159 = Match First String(2:w272, 3:w276) -> (0:w273:i32)  [unwired: 1 out]
                n160 = property on="Test Ring" class="Ring (strict)"("Value"=w273, "Strings []"=w272) -> ()  [unwired: 2 in, 2 out]
                n161 = property on="Test Ring" class="Ring (strict)"("Visible"=TRUE) -> ()  [unwired: 2 in, 2 out]
                n162 = property on="Test Slider" class="Slide (strict)"("Visible"=FALSE) -> ()  [unwired: 2 in, 2 out]
              }
              frame "White Balance  **" {
                n163 = Index Array(array=w283, index=1) -> (element=w284:cluster{string[]})
                n164 = call <vilib>:"NT Read String.vi"("Name"=w286) -> ("String"=w285:string)  [unwired: 9 in, 1 out]
                n165 = Unbundle(w284) -> (w281:string[])
                n166 = Match First String(2:w281, 3:w285) -> (0:w280:i32)  [unwired: 1 out]
                n167 = property on="Test Ring" class="Ring (strict)"("Value"=w280, "Strings []"=w281) -> ()  [unwired: 2 in, 2 out]
                n168 = property on="Test Ring" class="Ring (strict)"("Visible"=TRUE) -> ()  [unwired: 2 in, 2 out]
                n169 = property on="Test Slider" class="Slide (strict)"("Visible"=FALSE) -> ()  [unwired: 2 in, 2 out]
              }
              frame "Exposure  **" {
                n170 = Index Array(array=w292, index=2) -> (element=w293:cluster{string[]})
                n171 = call <vilib>:"NT Read String.vi"("Name"=w295) -> ("String"=w294:string)  [unwired: 9 in, 1 out]
                n172 = Unbundle(w293) -> (w289:string[])
                n173 = Match First String(2:w289, 3:w294) -> (0:w290:i32)  [unwired: 1 out]
                n174 = property on="Test Ring" class="Ring (strict)"("Value"=w290, "Strings []"=w289) -> ()  [unwired: 2 in, 2 out]
                n175 = property on="Test Ring" class="Ring (strict)"("Visible"=TRUE) -> ()  [unwired: 2 in, 2 out]
                n176 = property on="Test Slider" class="Slide (strict)"("Visible"=FALSE) -> ()  [unwired: 2 in, 2 out]
              }
              frame "Exposure Priority  **" {
                n177 = Index Array(array=w301, index=3) -> (element=w302:cluster{string[]})
                n178 = call <vilib>:"NT Read String.vi"("Name"=w304) -> ("String"=w303:string)  [unwired: 9 in, 1 out]
                n179 = Unbundle(w302) -> (w298:string[])
                n180 = Match First String(2:w298, 3:w303) -> (0:w299:i32)  [unwired: 1 out]
                n181 = property on="Test Ring" class="Ring (strict)"("Value"=w299, "Strings []"=w298) -> ()  [unwired: 2 in, 2 out]
                n182 = property on="Test Ring" class="Ring (strict)"("Visible"=TRUE) -> ()  [unwired: 2 in, 2 out]
                n183 = property on="Test Slider" class="Slide (strict)"("Visible"=FALSE) -> ()  [unwired: 2 in, 2 out]
              }
              frame "Color Enable  **" {
                n184 = Index Array(array=w310, index=4) -> (element=w311:cluster{string[]})
                n185 = call <vilib>:"NT Read String.vi"("Name"=w313) -> ("String"=w312:string)  [unwired: 9 in, 1 out]
                n186 = Unbundle(w311) -> (w307:string[])
                n187 = Match First String(2:w307, 3:w312) -> (0:w308:i32)  [unwired: 1 out]
                n188 = property on="Test Ring" class="Ring (strict)"("Value"=w308, "Strings []"=w307) -> ()  [unwired: 2 in, 2 out]
                n189 = property on="Test Ring" class="Ring (strict)"("Visible"=TRUE) -> ()  [unwired: 2 in, 2 out]
                n190 = property on="Test Slider" class="Slide (strict)"("Visible"=FALSE) -> ()  [unwired: 2 in, 2 out]
              }
              frame Default {
                n191 = property on="Test Ring" class="Ring (strict)"("Visible"=FALSE) -> ()  [unwired: 2 in, 2 out]
                n192 = property on="Test Slider" class="Slide (strict)"("Visible"=FALSE) -> ()  [unwired: 2 in, 2 out]
              }
              frame "Brightness  **", "Color Level  **", "Compression  **", "FPS  **", "Sharpness  **" {
                n193 = call <vilib>:"NT Read Number.vi"("Name"=w319) -> ("Numeric"=w318:dbl)  [unwired: 9 in, 1 out]
                n194 = local write "Test Slider"(w318) -> ()
                n195 = property on="Test Slider" class="Slide (strict)"("Visible"=TRUE, "Scale.Maximum"=100.0 ("Scale.Range:Maximum")) -> ()  [unwired: 2 in, 2 out]
                n196 = property on="Test Ring" class="Ring (strict)"("Visible"=FALSE) -> ()  [unwired: 2 in, 2 out]
              }
            }
          }
        }
        n197 = property on="Progress" class="Clust (strict)"("Visible"=FALSE) -> ()  [unwired: 2 in, 2 out]
      }
      event "Test Name": Mouse Enter {
        # "Populate the ring with the list of tests"
        n198 = event-data() -> ()  [unwired: 1 in, 1 out]
        n199 = call <vilib>:"NT Read String Array.vi"("Name"="/TestMode/TestList") -> ("String Array"=w328:string[])  [unwired: 9 in, 1 out]
        n200 = Build Array (concatenate)("Select the test to run...", w328) -> (w327:string[])
        n201 = property on="Test Name" class="Ring (strict)"("Strings []"=w327) -> ()  [unwired: 2 in, 2 out]
      }
      event "Test Name": Value Change {
        w331 = FALSE ("Visible")
        # "Tell the robot the test name to run"
        n202 = event-data() -> ("NewVal"=w335:u16)  [unwired: 1 in]
        n203 = property on="Test Name" class="Ring (strict)"() -> ("Strings []"=w336:string[])  [unwired: 2 in, 2 out]
        n204 = local write "Progress"(T7 {"Test Progress"=0, "Test Progress Text"=""} ("Progress")) -> ()
        n205 = Index Array(array=w336, index=w335) -> (element=w334:string)
        n206 = call <vilib>:"NT Write String.vi"("String"=w334, "Name"="/TestMode/TestName") -> ()  [unwired: 9 in, 1 out]
        n207 = property on="Progress" class="Clust (strict)"("Visible"=TRUE) -> ()  [unwired: 2 in, 2 out]
        n208 = property on="Motor" class="Clust (strict)"("Visible"=w331) -> ()  [unwired: 2 in, 2 out]
        n209 = property on="Test Slider" class="Slide (strict)"("Visible"=w331) -> ()  [unwired: 2 in, 2 out]
        n210 = property on="On/Off" class="Bool (strict)"("Visible"=w331) -> ()  [unwired: 2 in, 2 out]
        n211 = property on="Rev/Fwd" class="Clust (strict)"("Visible"=w331) -> ()  [unwired: 2 in, 2 out]
        n212 = property on="Test Ring" class="Ring (strict)"("Visible"=w331) -> ()  [unwired: 2 in, 2 out]
      }
      event "Select Auto": Mouse Enter {
        # "Populate the combo box with the list of autonomous options"
        n213 = event-data() -> ()  [unwired: 1 in, 1 out]
        n214 = call <vilib>:"NT Read String Array.vi"("Name"="Auto List") -> ("String Array"=w338:string[])  [unwired: 9 in, 1 out]
        n215 = property on="Select Auto" class="CmbBox"("Strings[]"=w338) -> ()  [unwired: 2 in, 2 out]
      }
      event "Select Auto": Value Change {
        # "User modified the Auto Selection. Write to NT variable so robot knows."
        n216 = event-data() -> ("NewVal"=w342:string)  [unwired: 1 in]
        n217 = call <vilib>:"NT Write String.vi"("String"=w342, "Name"="Auto Selector") -> ()  [unwired: 9 in, 1 out]
      }
      event "Command Selection": Value Change {
        # "Get the params and show in table"
        n218 = event-data() -> ("NewVal"=w349:i32)  [unwired: 1 in]
        n219 = property on="Command Selection" class="MCListbox (strict)"() -> ("ItemNames"=w347:string[][])  [unwired: 2 in, 2 out]
        n220 = call <vilib>:"WPI_DashboardUpdate Command Params.vi"("NewVal"=w349, "Commands"=w347, "Param Tbl"=w348) -> ()  [unwired: 8 in, 1 out]
      }
      event "Execute Command": Value Change {
        # "Started one, Unique ID holds\nresponse"
        n221 = event-data() -> ()  [unwired: 1 in, 1 out]
        n222 = property on="Command Selection" class="MCListbox (strict)"() -> ("ItemNames"=w361:string[][])  [unwired: 2 in, 2 out]
        n223 = Index Array(array=w361, index (row)="Command Selection", index (col)=0) -> (element=w359:string)
        n224 = call <vilib>:"Invoke Commands.vi"("Command Params"="Command Params", "Function Name"=w359) -> ("Params"=w355:u8, "Started"=w354:bool)  [unwired: 7 in, 1 out]
        n225 = Array Subset(array="Command Params", length (row)=w355) -> (w356:string[][])  [unwired: 3 in]
        n226 = Select(t="Executing" ("Cmd Status"), s=w354, f="" ("Cmd Status")) -> (s? t:f=→"Cmd Status":string)
      }
      event "Command Selection": Double Click {
        n227 = event-data() -> ("Row"=w371:i32)  [unwired: 1 in]
        n228 = property on="Command Selection" class="MCListbox (strict)"() -> ("ItemNames"=w374:string[][])  [unwired: 2 in, 2 out]
        n229 = local read "Command Params"() -> (w369:string[][])
        n230 = Index Array(array=w374, index (row)=w371, index (col)=0) -> (element=w372:string)
        n231 = call <vilib>:"Invoke Commands.vi"("Command Params"=w369, "Function Name"=w372) -> ("Params"=w368:u8, "Started"=w363:bool)  [unwired: 7 in, 1 out]
        n232 = Array Subset(array=w369, length (row)=w368) -> (w367:string[][])  [unwired: 3 in]
        n233 = Select(t="Executing" ("Cmd Status"), s=w363, f="" ("Cmd Status")) -> (s? t:f=w364:string)
        n234 = local write "Cmd Status"(w364) -> ()
      }
      event "CheckList": Double Click {
        # "Shift clears all"
        # "Update symbols on the listbox"
        n235 = event-data() -> ("PlatMods.Shift"=w377:bool, "Row"=w379:i32)  [unwired: 1 in]
        n236 = case shown="True" w377 {
          tunnel: w379 -> [w383 _]
          tunnel: 1 -> [w382 _]
          frame False {
            n237 = property on="CheckList" class="LstBox (strict)"() -> ("Item Symbols"=w381:i32[])  [unwired: 2 in, 2 out]
            n238 = Replace Array Subset(array=w381, new element=w382, index=w383) -> (w380:i32[])
            n239 = property on="CheckList" class="LstBox (strict)"("Item Symbols"=w380) -> ()  [unwired: 2 in, 2 out]
          }
          frame True {
            w384 = 0 ("Top Row")
            n240 = property on="CheckList" class="LstBox (strict)"() -> ("Number of Rows"=w386:u32)  [unwired: 2 in, 2 out]
            n241 = Initialize Array(0, w386) -> (w385:i32[])
            n242 = property on="CheckList" class="LstBox (strict)"("Top Row"=w384, "Value"=w384, "Item Symbols"=w385) -> ()  [unwired: 2 in, 2 out]
          }
        }
      }
      event "CheckList": Key Down {
        # "Update symbols on the listbox\nLeft and right keys check and uncheck"
        n243 = event-data() -> ("VKey"=w391:T23)  [unwired: 1 in]
        n244 = case shown="\"Left\", \"Right\"" w391 {
          selector: w391 -> [w396 _]
          tunnel: eventvkey."Left" ("VKey") -> [w394 _]
          frame "Left", "Right" {
            n245 = Equal?(x=w394, y=w396) -> (x = y?=w395:bool)
            n246 = Select(t=0, s=w395, f=1) -> (s? t:f=w397:i32)
            n247 = property on="CheckList" class="LstBox (strict)"() -> ("Item Symbols"=w400:i32[])  [unwired: 2 in, 2 out]
            n248 = Replace Array Subset(array=w400, new element=w397, index="CheckList") -> (w399:i32[])
            n249 = property on="CheckList" class="LstBox (strict)"("Item Symbols"=w399) -> ()  [unwired: 2 in, 2 out]
          }
          frame Default {
          }
        }
      }
      event "DB Camera Config": Value Change {
        # "Show or hide the cluster of controls, store in ini file"
        n250 = event-data() -> ("NewVal"=w405:bool)  [unwired: 1 in]
        n251 = case shown="False" w405 {
          tunnel: w404 -> [w414 _]
          tunnel: [w407 w425] -> w403
          tunnel: w402 -> [w406 w425]
          frame False {
            w421 = "Camera"
            w424 = FALSE ("Visible")
            n252 = local read "Camera Settings"() -> (w413:T2)
            n253 = Index Array(array=w414) -> (element=w417:cluster{string[]})  [unwired: 1 in]
            n254 = Unbundle(w413) -> ("Frame Rate"=w412:i32, "Compression"=w411:i32, "Size"=w415:u16)
            n255 = Unbundle(w417) -> (w416:string[])
            n256 = Index Array(array=w416, index=w415) -> (element=w410:string)
            n257 = call-poly <vilib>:"Write Key.vi"("section"=w421, "value"=w410, "key"="Size", "refnum"=w406) -> ("refnum out"=w423:T21)  [unwired: 2 in, 5 out]
            n258 = call-poly <vilib>:"Write Key.vi"("section"=w421, "value"=w412, "key"="FrameRate", "refnum"=w423) -> ("refnum out"=w422:T21)  [unwired: 1 in, 6 out]
            n259 = property on="Camera Settings" class="Clust (strict)"("Visible"=w424) -> ()  [unwired: 2 in, 2 out]
            n260 = local write "DB Camera Config"(w424) -> ()
            n261 = call-poly <vilib>:"Write Key.vi"("section"=w421, "value"=w411, "key"="Compression", "refnum"=w422) -> ("refnum out"=w408:T21)  [unwired: 1 in, 6 out]
            n262 = call <vilib>:"Close Config Data.vi"("refnum"=w408) -> ("file path"=w409:path)  [unwired: 2 in, 8 out]
            n263 = call <vilib>:"Open Config Data.vi"("configuration file path"=w409) -> ("refnum"=w407:T21)  [unwired: 8 in, 2 out]
          }
          frame True {
            n264 = property on="Camera Settings" class="Clust (strict)"("Visible"=TRUE) -> ()  [unwired: 2 in, 2 out]
          }
        }
      }
      event "Camera Settings": Value Change {
        # "Update summary string when any elements of DB camera change"
        n265 = event-data() -> ("NewVal"=w439:T2)  [unwired: 1 in]
        n266 = Index Array(array=w435) -> (element=w434:cluster{string[]})  [unwired: 1 in]
        n267 = Unbundle(w439) -> ("Frame Rate"=w430:i32, "Compression"=w429:i32, "Size"=w432:u16)
        n268 = Unbundle(w434) -> (w433:string[])
        n269 = Index Array(array=w433, index=w432) -> (element=w431:string)
        n270 = Format Into String(format string="%s   %dfps   %d%%", w431, w430, w429) -> (resulting string=w436:string)  [unwired: 2 in, 1 out]
        n271 = Build Array(w436) -> (w437:string[])
        n272 = property on="DB Camera Config" class="Bool (strict)"("Strings [4]"=w437) -> ()  [unwired: 2 in, 2 out]
      }
      event "Motor.Enable": Value Change {
        # "When the test mode otor enable helper is set, update that\ntree row item's value"
        n273 = event-data() -> ("NewVal"=w446:bool)  [unwired: 1 in]
        n274 = Unbundle("Motor") -> ("Value"=w445:dbl)  [unwired: 1 out]
        n275 = Select(t=w445, s=w446, f=0.0) -> (s? t:f=w443:dbl)
        n276 = call <vilib>:"NT Write Number.vi"("Numeric"=w443, "Name"=w442) -> ()  [unwired: 9 in, 1 out]
      }
      event "Test Slider": Value Change {
        # "When the test mode slider helper is set, update that\ntree row item's value"
        n277 = event-data() -> ("NewVal"=w450:dbl)  [unwired: 1 in]
        n278 = call <vilib>:"NT Write Number.vi"("Numeric"=w450, "Name"=w451) -> ()  [unwired: 9 in, 1 out]
      }
      event "On/Off": Value Change {
        # "When the test mode on/off helper value is set, update that\ntree row item's value"
        n279 = event-data() -> ("NewVal"=w456:bool)  [unwired: 1 in]
        n280 = Boolean To (0,1)(Boolean=w456) -> (0, 1=w455:i16)
        n281 = call <vilib>:"NT Write Number.vi"("Numeric"=w455, "Name"=w454) -> ()  [unwired: 9 in, 1 out]
      }
      event "Rev/Fwd": Value Change {
        # "When the test mode helper value for relays is set, update that\ntree row item's value"
        n282 = event-data() -> ("NewVal.Forward"=w465:bool, "NewVal.Reverse"=w464:bool)  [unwired: 1 in]
        n283 = Boolean To (0,1)(Boolean=w465) -> (0, 1=w461:i16)
        n284 = Boolean To (0,1)(Boolean=w464) -> (0, 1=w463:i16)
        n285 = Negate(x=w463) -> (-x=w462:i16)
        n286 = Add(x=w461, y=w462) -> (x+y=w460:i16)
        n287 = call <vilib>:"NT Write Number.vi"("Numeric"=w460, "Name"=w459) -> ()  [unwired: 9 in, 1 out]
      }
      event "Test Ring": Value Change {
        # "When a test mode helper value is selected from the ring,\nset the tree item's variable to the string value"
        n288 = event-data() -> ("NewVal"=w470:u16)  [unwired: 1 in]
        n289 = property on="Test Ring" class="Ring (strict)"() -> ("Strings []"=w471:string[])  [unwired: 2 in, 2 out]
        n290 = Index Array(array=w471, index=w470) -> (element=w469:string)
        n291 = call <vilib>:"NT Write String.vi"("String"=w469, "Name"=w468) -> ()  [unwired: 9 in, 1 out]
      }
      event "Rec Mode": Value Change {
        # "Update globals for recording mode and path to read log from.\nClear when logging and let NetworkTables set path for vision to\nuse."
        n292 = event-data() -> ("NewVal"=w483:enum32{"Stop", "Record", "Playback"})  [unwired: 1 in]
        n293 = global write "WPI_DashboardLogging Global.vi" "Logging Filename"(path "") -> ()
        n294 = global write "WPI_DashboardLogging Global.vi" "Recording"(w483) -> ()
        n295 = case shown="\"Playback\"" w483 {
          tunnel: w482 -> [_ w485 w494]
          tunnel: [_ _ w493] -> w479
          tunnel: [_ _ w492] -> _
          tunnel: w477 -> [_ _ w490]
          tunnel: cluster{i32, i32} {-250, 170} -> [_ _ w489]
          tunnel: [_ _ T24 {"Image Size"=TRUE, "Image Type"=TRUE, "Pixel Value"=TRUE, "ROI Information"=TRUE, "Zoom Factor"=FALSE} ("Image Information Shown:All Elements")] -> w475
          tunnel: [_ _ TRUE ("Zoom Factor")] -> w474
          tunnel: w473 -> [_ _ w486]
          frame Default {
          }
          frame "Stop", "Record" {
            # "Place Window too"
            n296 = invoke class="VI" method="FP.Close"(reference=w485) -> (reference out=w484:refnum<vi>)  [unwired: 2 in, 2 out]
            n297 = invoke class="VI" method="Abort VI"(reference=w484) -> ()  [unwired: 2 in, 3 out]
          }
          frame "Playback" {
            n298 = call "Open Playback Panel.vi"("Offset"=w489, "DB VI Ref"=w490, "Playback in"=w494) -> ("Playback out"=w491:refnum<vi>)  [unwired: 8 in]
            n299 = register-events(w491, w486) -> (reference out=w493:refnum<event-registration>, error out=w492:errorcluster)  [unwired: 2 in]
          }
        }
        n300 = property on="Camera Image" class="ImageControl"("Image Information Shown"=w475, "Image Information Visible"=w474) -> ()  [unwired: 2 in, 2 out]
        n301 = call <vilib>:"WPI_DashboardNT Log FieldName Cache.vi"("Operation"=enum16{"Lookup/Add", "Index", "Clear"}."Clear") -> ()  [unwired: 8 in, 3 out]
      }
      event Panel Close {
        w496 = enum32{"Stop", "Record", "Playback"}."Stop" ("Rec Mode")
        # "Playback window has been closed, abort"
        n302 = event-data() -> ()  [unwired: 1 in, 4 out]
        n303 = local write "Rec Mode"(w496) -> ()
        n304 = global write "WPI_DashboardLogging Global.vi" "Recording"(w496) -> ()
      }
      event Panel Close {
        # "Abort playback window and ourself"
        n305 = event-data() -> ()  [unwired: 1 in, 4 out]
        n306 = invoke class="VI" method="FP.Close"(reference=w502) -> (reference out=w501:refnum<vi>)  [unwired: 2 in, 2 out]
        n307 = invoke class="VI" method="Abort VI"(reference=w501) -> (error out=w500:errorcluster)  [unwired: 2 in, 2 out]
        n308 = invoke class="VI" method="Abort VI"(error in=w500) -> ()  [unwired: 2 in, 3 out]
      }
      event User Event {
        n309 = event-data() -> ("IDs"=w510:cluster{"RPC field ID":u16, "Unique ID":u16}, "String"=w509:string)  [unwired: 1 in]
        n310 = Bundle("IDs"=w510, "String"=w509) -> (w508:T9)  [unwired: 1 in]
        n311 = call <vilib>:"Retrieve RPC Response.vi"("RPC Response"=w508) -> ("Output"=w505:string[][])  [unwired: 10 in]
        n312 = Build Array (concatenate)(w503, w505) -> (w504:string[][])
        n313 = local write "Command Params"(w504) -> ()
        n314 = local write "Cmd Status"("" ("Cmd Status")) -> ()
      }
      event "Vision": Value Change {
        # "Enable/Disable Compression slider.\nHW USB is hard-coded into the camera"
        n315 = event-data() -> ("NewVal"=w517:u16)  [unwired: 1 in]
        n316 = Equal?(x=w517, y=u32 2 ("milliseconds to wait")) -> (x = y?=w515:bool)
        n317 = Select(t=T25."Disabled and Grayed Out" ("Disabled"), s=w515, f=T25."Enabled" ("Disabled")) -> (s? t:f=w512:T25)
        n318 = property on="Compression" class="Slide (strict)"("DisabledEnum"=w512) -> ()  [unwired: 2 in, 2 out]
      }
      event "Tree": Double Click {
        n319 = event-data() -> ("PlatMods"=w522:T28, "Tag"=w521:string)  [unwired: 1 in]
        n320 = Unbundle(w522) -> ("Shift"=w520:bool)  [unwired: 4 out]
        n321 = Not(x=w520) -> (.not. x?=w519:bool)
        n322 = call <vilib>:"NT Update Persistence.vi"("Persistence"=w519, "Name"=w521) -> ()  [unwired: 9 in, 1 out]
      }
    }
  }
  n323 = while {
    tunnel: w47 -> [w526]
    i -> [w529]
    stop <- FALSE stop-if-true
    n324 = Wait (ms)(milliseconds to wait=u32 100) -> ()  [unwired: 1 out]
    n325 = case shown="\"Playback\"" "Rec Mode" {
      tunnel: w529 -> [_ _ w544]
      tunnel: [u32 2829099 ("Base Color") u32 11141120 ("Target Color") w533] -> w525
      frame "Stop", Default {
        # "Reset the color, extra updates don't cost much"
      }
      frame "Record" {
      }
      frame "Playback" {
        # "Playback"
        n326 = Quotient & Remainder(x=w544, y=u32 50 ("milliseconds to wait")) -> (x-y*floor(x/y)=w540:u32)  [unwired: 1 out]
        n327 = Divide(x=w540, y=u32 50 ("milliseconds to wait")) -> (x/y=w537:dbl)
        n328 = Multiply(x=6.283185307179586, y=w537) -> (x*y=w542:dbl)
        n329 = Sine(x=w542) -> (sin(x)=w541:dbl)
        n330 = Absolute Value(x=w541) -> (abs(x)=w534:dbl)
        n331 = call "Interpolate RGB Color.vi"("Proportion"=w534, "Target Color"=u32 30976, "Base Color"=u32 2829099) -> ("Result Color"=w533:u32)  [unwired: 8 in]
      }
    }
    n332 = property class="Pane"(reference=w526, "PaneColor"=w525) -> ()  [unwired: 1 in, 2 out]
  }
  n333 = local write "Dashboard Tab"(T1."Drive" ("Dashboard Tab")) -> ()
  n334 = property on="On/Off" class="Bool (strict)"("Visible"=w15) -> ()  [unwired: 2 in, 2 out]
  n335 = property on="Motor" class="Clust (strict)"("Visible"=w15) -> ()  [unwired: 2 in, 2 out]
  n336 = property on="Progress" class="Clust (strict)"("Visible"=w15) -> ()  [unwired: 2 in, 2 out]
  n337 = property on="Test Ring" class="Ring (strict)"("Visible"=w15) -> ()  [unwired: 2 in, 2 out]
  n338 = property on="Rev/Fwd" class="Clust (strict)"("Visible"=w15) -> ()  [unwired: 2 in, 2 out]
  n339 = property on="Camera Settings" class="Clust (strict)"("Visible"=w15) -> ()  [unwired: 2 in, 2 out]
  n340 = while {
    tunnel: u16 1741 ("timeout ms (25000)") -> [w546]
    stop <- FALSE stop-if-true
    n341 = TCP Create Listener(10:w546) -> (0:w545:errorcluster, 3:w547:refnum<k5>)  [unwired: 4 in, 1 out]
    n342 = case shown="No Error" w545 {
      selector: w545 -> [w549 _]
      tunnel: w547 -> [w550 _]
      frame No Error {
        n343 = while {
          tunnel: w550 -> [w553]
          tunnel: w549 -> [w552]
          stop <- FALSE stop-if-true
          n344 = TCP Wait On Listener(8:w552, 11:w553) -> (0:w554:errorcluster, 4:w555:refnum<k5>)  [unwired: 2 in, 3 out]
          n345 = local write "TCP"(w555) -> ()
          n346 = case shown="No Error" w554 {
            frame No Error {
            }
            frame Error {
              n347 = Wait (ms)(milliseconds to wait=u32 1000) -> ()  [unwired: 1 out]
            }
          }
        }
      }
      frame Error {
        n348 = Wait (ms)(milliseconds to wait=u32 1000) -> ()  [unwired: 1 out]
      }
    }
  }
  n349 = local write "DB Camera Config"(w15) -> ()
  n350 = local write "Command Params"(string[][] [] ("Command Params")) -> ()
  n351 = global write "WPI_DashboardLogging Global.vi" "Recording"(w41) -> ()
  n352 = local write "Command Selection"(u16 0 ("milliseconds to wait")) -> ()
  n353 = local write "Rec Mode"(w41) -> ()
